vi "Read Roles.vi"(8 "error in (no error)":errorcluster, 11 "PassToStriker in":refnum<class "PassToStriker.lvclass">) -> (0 "error out":errorcluster, 2 "Role":T1, 3 "PassToStriker out":refnum<class "PassToStriker.lvclass">)   [LabVIEW 2018, in "PassToStriker.lvclass"]
uses:
  PassToStriker.lvclass
  PassKickerRole_class/PassKickerRole.lvclass
  PassReceiverRole_class/PassReceiverRole.lvclass
  PassObserverRole_class/PassObserverRole.lvclass
  PassToStriker.lvclass/PassToStriker.ctl
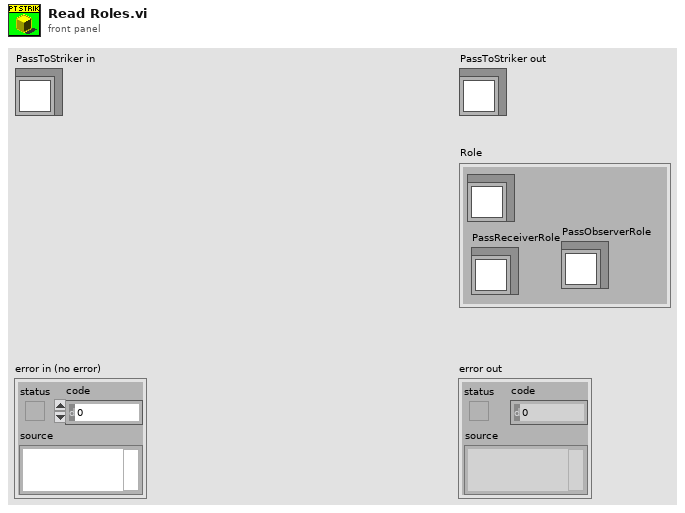
[diagram p1: front panel]
types:
  T1 = cluster{"PassKickerRole":refnum<class "PassKickerRole.lvclass">, "PassReceiverRole":refnum<class "PassReceiverRole.lvclass">, "PassObserverRole":refnum<class "PassObserverRole.lvclass">}
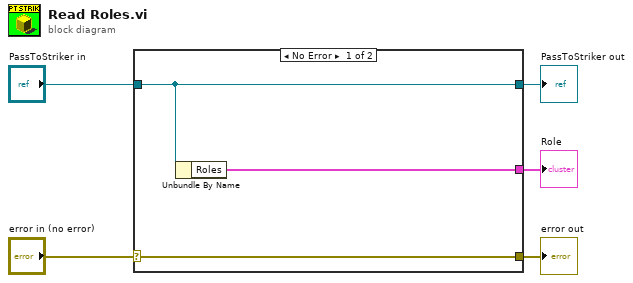
[diagram p0: block diagram]
diagram:
  n1 = case shown="No Error" "error in (no error)" {
    selector: "error in (no error)" -> [w8 w9]
    tunnel: [w8 w9] -> w4
    tunnel: [w7 w10] -> w2
    tunnel: "PassToStriker in" -> [w7 w10]
    tunnel: [w6 _] -> w1
    frame No Error {
      n2 = Unbundle By Name(w7) -> ("Roles"=w6:T1)
    }
    frame Error {
    }
  }
  "error out" <- w4
  "PassToStriker out" <- w2
  "Role" <- w1
